vi "Read configuration.vi"(8 "error in (no error)":errorcluster, 11 "Scope Channel":refnum<class "Scope Channel.lvclass">) -> (0 "error out":errorcluster, 2 "configuration":refnum<class "CEF_serializable configuration.lvclass">, 3 "Scope Channel out":refnum<class "Scope Channel.lvclass">)   [LabVIEW 2025, in "Scope.lvlib" / "Scope Channel.lvclass"]
uses:
  Scope Channel.lvclass
  Users/Public/Documents/Sandia National Labs/TSS Plugin/CEF.lvlibp/serializable configuration/CEF_serializable configuration.lvclass
  Scope Channel.lvclass/Scope Channel.ctl
  Scope Channel configuration/Scope Channel configuration.lvclass
  C:/Users/Public/Documents/Sandia National Labs/TSS Plugin/CEF.lvlibp/serializable configuration/CEF_serializable configuration.lvclass
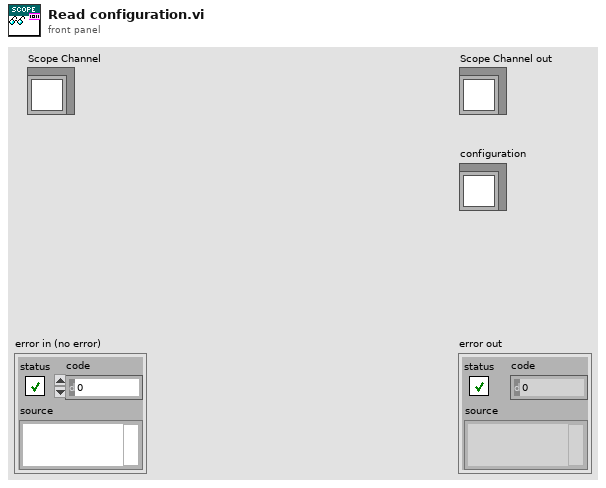
[diagram p1: front panel]
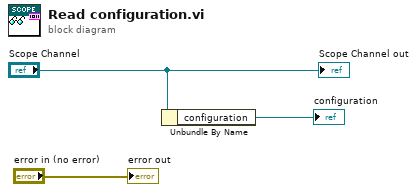
[diagram p0: block diagram]
diagram:
  n1 = Unbundle By Name("Scope Channel") -> ("configuration"=→"configuration":refnum<class "Scope Channel configuration.lvclass">)
  "error out" <- "error in (no error)"
  "Scope Channel out" <- "Scope Channel"
